vi "Amplitude.vi"() -> ()   [LabVIEW 2018]
uses:
  <vilib>/measure/NI_MABase.lvlib
panel:
  out "Positive Peak":dbl
  out "Negative Peak":dbl
  out "signal out":waveform(dbl)(graph)
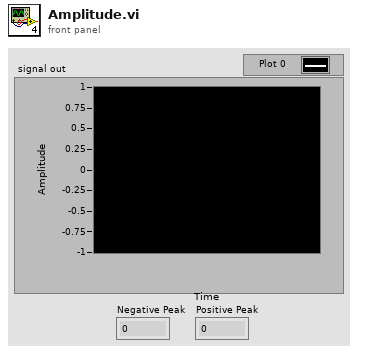
[diagram p1: front panel]
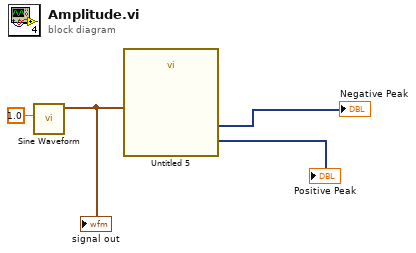
[diagram p0: block diagram]
diagram:
  n1 = call <vilib>:"Sine Waveform.vi"("amplitude"=1.0) -> ("signal out"=w3:waveform(dbl))  [unwired: 9 in, 1 out]
  "signal out" <- w3
  n2 = call "Untitled 5.vi"("Signals"=w3) -> ("Negative Peak"=→"Negative Peak":dynamicdata, "Positive Peak"=→"Positive Peak":dynamicdata)  [unwired: 12 in, 1 out]
